vi "Create LV Class in Library.vi"(8 "error in":errorcluster, 9 "new class folder":path, 10 "new class file name":string, 11 "library reference in":refnum<vi>) -> (0 "error out":errorcluster, 2 "class reference":refnum<vi>, 3 "library reference out":refnum<vi>)   [LabVIEW 2019, in "gRPC Template Creation Utility.lvlib"]
uses:
  gRPC Template Creation Utility.lvlib
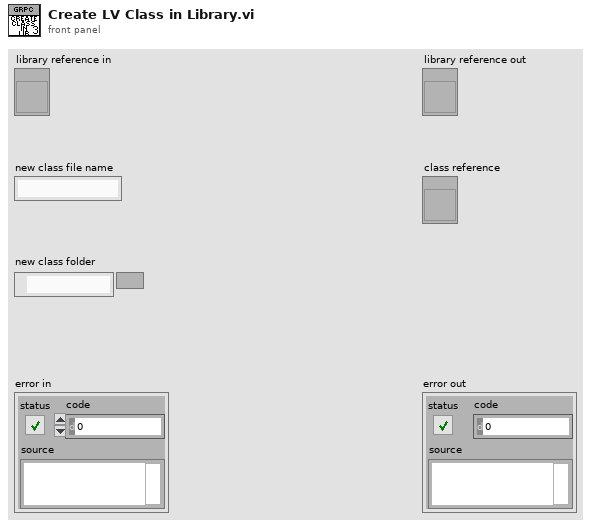
[diagram p1: front panel]
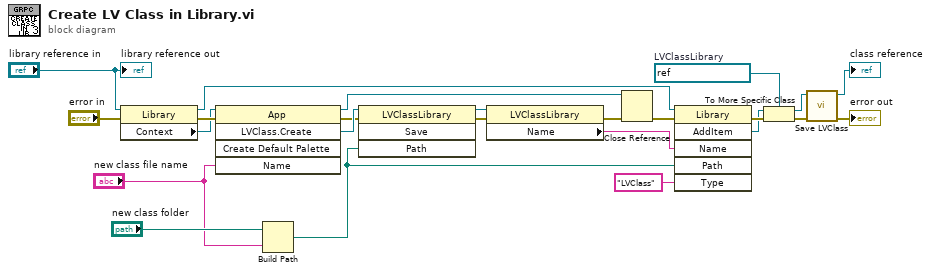
[diagram p0: block diagram]
diagram:
  w4 = refnum<vi> refnum  # LVClassLibrary
  n1 = property class="Library"(reference="library reference in", error in="error in") -> (reference out=w18:refnum<vi>, error out=w24:errorcluster, "Context"=w21:refnum<vi>)
  n2 = invoke class="App" method="LVClass.Create"(reference=w21, error in=w24, "Name"="new class file name") -> (reference out=w14:refnum<vi>, error out=w19:errorcluster, "LVClass.Create"=w20:refnum<vi>)  [unwired: 2 in, 2 out]
  n3 = Build Path(base path="new class folder", name or relative path="new class file name") -> (appended path=w8:path)
  n4 = invoke class="LVClassLibrary" method="Save"(reference=w20, error in=w19, "Path"=w8) -> (reference out=w16:refnum<vi>, error out=w11:errorcluster)  [unwired: 1 in, 2 out]
  n5 = property class="LVClassLibrary"(reference=w16, error in=w11) -> (error out=w13:errorcluster, "Name"=w15:string)  [unwired: 1 out]
  n6 = Close Reference(reference=w14, error in (no error)=w13) -> (error out=w12:errorcluster)
  n7 = invoke class="Library" method="AddItem"(reference=w18, error in=w12, "Name"=w15, "Path"=w8, "Type"="LVClass") -> (error out=w6:errorcluster, "AddItem"=w5:refnum<vi>)  [unwired: 1 in, 4 out]
  n8 = To More Specific Class(target class=w4, reference=w5, error in=w6) -> (specific class reference=w2:refnum<vi>, error out=w3:errorcluster)
  n9 = call "Save LVClass.vi"("error in (no error)"=w3, "LVClassLibrary in"=w2) -> ("error out"=→"error out":errorcluster, "LVClassLibrary out"=→"class reference":refnum<vi>)  [unwired: 8 in]
  "library reference out" <- "library reference in"
